vi "split PID parameters.vi"(2 "string":string) -> (7 "PID out":cluster{"Kp":dbl, "Ki":dbl, "Kd":dbl})   [LabVIEW 2011]
panel:
  # "Split PID parameters"
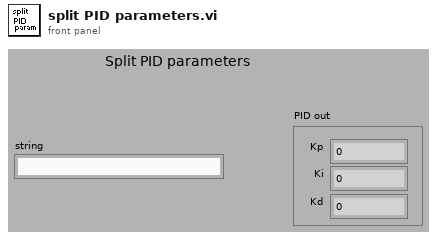
[diagram p1: front panel]
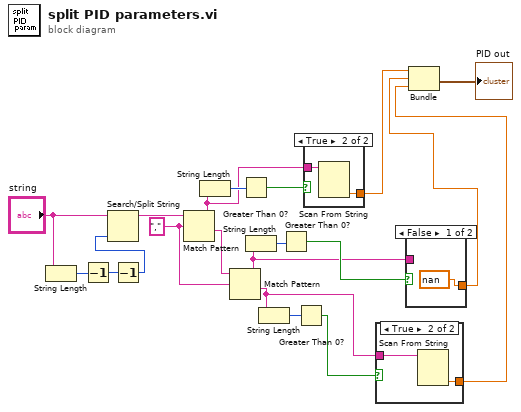
[diagram p0: block diagram]
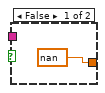
[diagram p2: hidden frame]
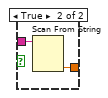
[diagram p3: hidden frame]
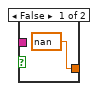
[diagram p4: hidden frame]
diagram:
  w20 = "," ("regular expression")
  n1 = String Length(string="string") -> (length=w5:i32)
  n2 = Decrement(x=w5) -> (x-1=w4:i32)
  n3 = Decrement(x=w4) -> (x-1=w1:i32)
  n4 = Search/Split String(string="string", offset (0)=w1) -> (substring before match=w2:string)  [unwired: 1 in, 2 out]
  n5 = Match Pattern(string=w2, regular expression=w20) -> (before substring=w16:string, after substring=w19:string)  [unwired: 1 in, 2 out]
  n6 = String Length(string=w16) -> (length=w18:i32)
  n7 = Match Pattern(string=w19, regular expression=w20) -> (before substring=w12:string, after substring=w6:string)  [unwired: 1 in, 2 out]
  n8 = Greater Than 0?(x=w18) -> (x > 0?=w17:bool)
  n9 = String Length(string=w12) -> (length=w15:i32)
  n10 = String Length(string=w6) -> (length=w14:i32)
  n11 = Greater Than 0?(x=w15) -> (x > 0?=w13:bool)
  n12 = Greater Than 0?(x=w14) -> (x > 0?=w11:bool)
  n13 = case shown="True" w17 {
    tunnel: w16 -> [_ w23]
    tunnel: [nan w22] -> w9
    frame False {
    }
    frame True {
      n14 = Scan From String(input string=w23) -> (output 1=w22:dbl)  [unwired: 4 in, 3 out]
    }
  }
  n15 = case shown="True" w11 {
    tunnel: w6 -> [_ w26]
    tunnel: [nan w25] -> w8
    frame False {
    }
    frame True {
      n16 = Scan From String(input string=w26) -> (output 1=w25:dbl)  [unwired: 4 in, 3 out]
    }
  }
  n17 = case shown="False" w13 {
    tunnel: w12 -> [_ w29]
    tunnel: [nan w28] -> w10
    frame False {
    }
    frame True {
      n18 = Scan From String(input string=w29) -> (output 1=w28:dbl)  [unwired: 4 in, 3 out]
    }
  }
  n19 = Bundle(w9, w10, w8) -> (→"PID out":cluster{dbl, dbl, dbl})  [unwired: 1 in]
